vi "write pockels cell task.vi"(8 "error in (no error)":errorcluster, 11 "Waveform in":refnum<class "Waveform.lvclass">) -> (0 "error out":errorcluster, 3 "Waveform out":refnum<class "Waveform.lvclass">)   [LabVIEW 2012, in "Waveform.lvclass"]
uses:
  Waveform.lvclass
  Waveform.lvclass/Waveform.ctl
  <vilib>/DAQmx/write.llb/DAQmx Write (Analog DBL 1Chan 1Samp).vi
  <vilib>/DAQmx/miscellaneous.llb/DAQmx Fill In Error Info.vi
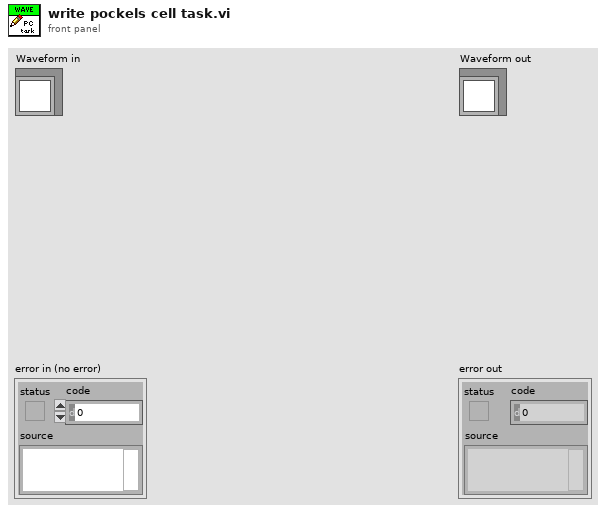
[diagram p1: front panel]
types:
  T1 = typedef "PC_wavelength.ctl" = dbl
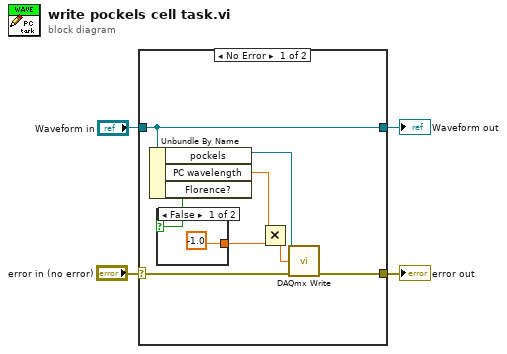
[diagram p0: block diagram]
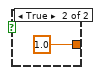
[diagram p2: hidden frame]
diagram:
  n1 = case shown="No Error" "error in (no error)" {
    selector: "error in (no error)" -> [w10 w16]
    tunnel: [w12 w16] -> w3
    tunnel: [w11 w15] -> w1
    tunnel: "Waveform in" -> [w11 w15]
    frame No Error {
      n2 = Unbundle By Name(w11) -> ("pockels"=w9:refnum<k21>, "PC wavelength"=w6:T1, "Florence?"=w8:bool)
      n3 = case shown="False" w8 {
        tunnel: [-1.0 1.0] -> w7
        frame False {
        }
        frame True {
        }
      }
      n4 = Multiply(x=w6, y=w7) -> (x*y=w5:T1)
      n5 = call-poly <vilib>:"DAQmx Write.vi"("task/channels in"=w9, "data"=w5, "error in"=w10) -> ("error out"=w12:errorcluster)  [unwired: 10 in, 2 out]
    }
    frame Error {
    }
  }
  "error out" <- w3
  "Waveform out" <- w1
